vi "HW Stop.vi"(8 "error in (no error)":errorcluster) -> (0 "error out":errorcluster)   [LabVIEW 2020]
uses:
  Global Variables/General Globals.vi
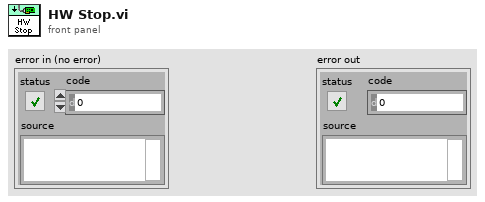
[diagram p1: front panel]
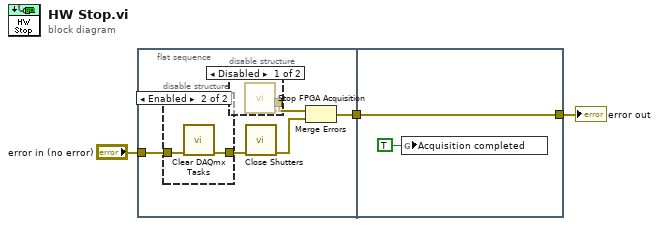
[diagram p0: block diagram]
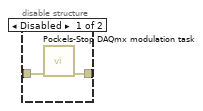
[diagram p3: hidden frame]
diagram:
  n1 = flat-sequence {
    tunnel: "error in (no error)" -> [w4]
    tunnel: [w8] -> w1
    tunnel: [w15] -> w3
    tunnel: w1 -> [w15]
    frame #0 {
      n2 = disable-structure shown="Enabled" {
        disable-tunnel: [w11 w12] -> w5
        disable-tunnel: w4 -> [w10 w13]
        frame Disabled {
          n3 = call "Pockels-Stop DAQmx modulation task.vi"("error in"=w10) -> ("error out"=w11:errorcluster)  [unwired: 10 in]
        }
        frame Enabled {
          n4 = call "Clear DAQmx Tasks.vi"("error in (no error)"=w13) -> ("error out"=w12:errorcluster)  [unwired: 10 in]
        }
      }
      n5 = disable-structure shown="Disabled" {
        disable-tunnel: [w9 _] -> w7
        frame Disabled {
          n6 = call "Stop FPGA Acquisition.vi"() -> ("Error Out"=w9:errorcluster)  [unwired: 10 in, 1 out]
        }
        frame Enabled {
        }
      }
      n7 = call "Close Shutters.vi"("error in (no error)"=w5) -> ("error out (no error)"=w6:errorcluster)  [unwired: 10 in]
      n8 = Merge Errors(w7, w6) -> (w8:errorcluster)
    }
    frame #1 {
      n9 = global write "General Globals.vi" "Acquisition completed"(TRUE ("Acquisition completed")) -> ()
    }
  }
  "error out" <- w3
